vi "Set Scene Item Rotation.vi"(6 "Rotation Deg":dbl, 8 "error in (no error)":errorcluster, 9 "Scene Item ID":i32, 10 "Scene Name":string, 11 "OBS in":refnum<class "OBS.lvclass">) -> (0 "error out":errorcluster, 3 "OBS out":refnum<class "OBS.lvclass">)   [LabVIEW 2020, in "obs-websocket.lvlib" / "OBS.lvclass"]
uses:
  OBS.lvclass
  OBS.lvclass/OBS.ctl
  JSONRequest/JSONRequest.lvclass
  REmptyResponse/REmptyResponse.lvclass
  C:/dev/lv20CE/relink/lv-obs-websocket/obs-websocket/Response/Response.lvclass
  C:/dev/lv20CE/relink/lv-obs-websocket/obs-websocket/Server Message/Server Message.lvclass
  C:/dev/lv20CE/relink/lv-obs-websocket/obs-websocket/Message/Message.lvclass
  C:/dev/lv20CE/relink/lv-promises/Promises/Value/Value.lvclass
  C:/dev/lv20CE/relink/lv-obs-websocket/obs-websocket/REmptyResponse/REmptyResponse.lvclass
  C:/dev/lv20CE/relink/lv-obs-websocket/obs-websocket/Request/Request.lvclass
  C:/dev/lv20CE/relink/lv-obs-websocket/obs-websocket/Client Message/Client Message.lvclass
  C:/dev/lv20CE/relink/lv-obs-websocket/obs-websocket/JSONRequest/JSONRequest.lvclass
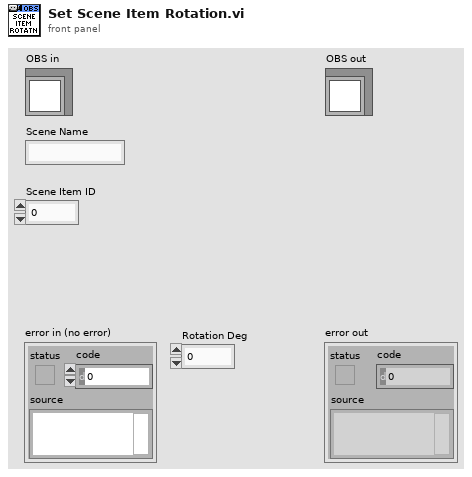
[diagram p1: front panel]
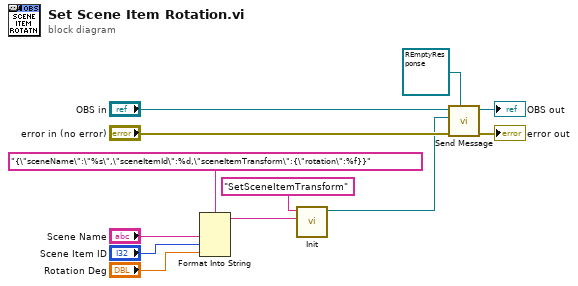
[diagram p0: block diagram]
diagram:
  n1 = Format Into String(format string="{\"sceneName\":\"%s\",\"sceneItemId\":%d,\"sceneItemTransform\":{\"rotation\":%f}}", "Scene Name", "Scene Item ID", "Rotation Deg") -> (resulting string=w7:string)  [unwired: 2 in, 1 out]
  n2 = call "Init.vi"("JSON"=w7, "Type"="SetSceneItemTransform") -> ("JSONRequest out"=w1:refnum<class "JSONRequest.lvclass">)  [unwired: 8 in, 1 out]
  n3 = call "Send Message.vi"("Response Type (None)"=refnum<class "REmptyResponse.lvclass"> refnum ("obs-websocket-lv.lvlib:REmptyResponse.lvclass"), "error in (no error)"="error in (no error)", "Client Message"=w1, "OBS in"="OBS in") -> ("error out"=→"error out":errorcluster, "OBS out"=→"OBS out":refnum<class "OBS.lvclass">)  [unwired: 4 in, 2 out]
